vi "Add Item to Tree.vi"(8 "error in (no error)":errorcluster, 10 "Polymorphic VI Type in":refnum<class "Polymorphic VI Type.lvclass">, 11 "Tree Ref in":refnum<vi>) -> (0 "error out":errorcluster, 1 "Added Tag":string, 2 "Polymorphic VI Type out":refnum<class "Polymorphic VI Type.lvclass">, 3 "Tree Ref out":refnum<vi>)   [LabVIEW 2020, in "Peek Window.lvlib" / "Polymorphic VI Type.lvclass"]
uses:
  Polymorphic VI Type.lvclass
  D:/Code/VI-Peek/source/Peek Window/VI Types/Standard VI Type/Standard VI Type.lvclass
  Symbols Enum.ctl
  Standard VI Type/Standard VI Type.lvclass/Standard VI Type.ctl
  Standard VI Type/Read Full Qualified Name.vi
  Polymorphic VI Type.lvclass/Polymorphic VI Type.ctl
  Peek Window.lvlib
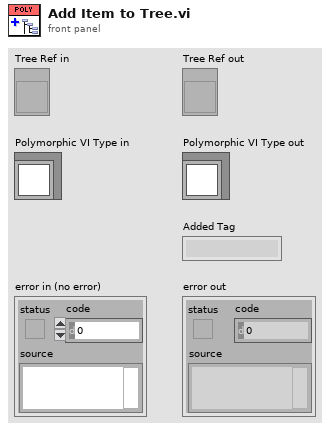
[diagram p1: front panel]
types:
  T1 = typedef "Peek Window.lvlib/Symbols Enum.ctl" = enum16{"<Blank>", "Below Here Glyph", "VI", "Dynamic Dispatch VI", "Malleable VI", "Polymorphic VI", "Missing VI", "Express VI"}
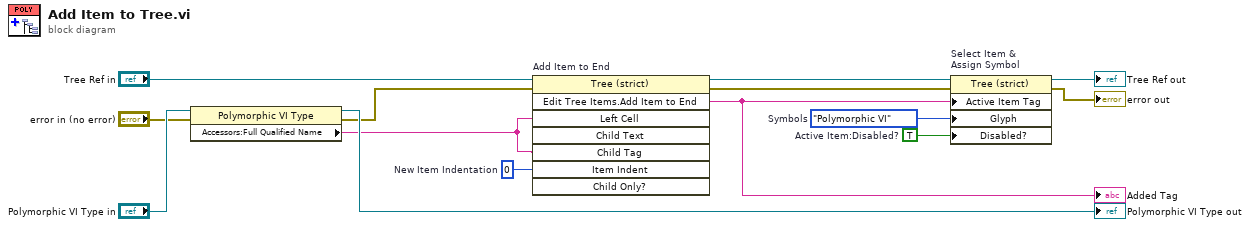
[diagram p0: block diagram]
diagram:
  w1 = TRUE  # Active Item:Disabled?
  w13 = Symbols_Enum."Polymorphic VI"  # Symbols
  w14 = 0  # New Item Indentation
  n1 = property class="Polymorphic VI Type"(reference="Polymorphic VI Type in", error in="error in (no error)") -> (reference out=→"Polymorphic VI Type out":refnum<class "Polymorphic VI Type.lvclass">, error out=w3:errorcluster, "Accessors:Full Qualified Name"=w2:string)
  n2 = invoke on="Add Item to End" class="Tree (strict)" method="Edit Tree Items.Add Item to End"(reference="Tree Ref in", error in=w3, "Left Cell"=w2, "Child Tag"=w2, "Item Indent"=w14) -> (reference out=w12:refnum<vi>, error out=w9:errorcluster, "Edit Tree Items:Add Item to End"=w7:string)  [unwired: 3 in, 5 out]
  "Added Tag" <- w7
  n3 = property on="Select Item &\nAssign Symbol" class="Tree (strict)"(reference=w12, error in=w9, "Active Item Tag"=w7, "Glyph"=w13, "Disabled?"=w1) -> (reference out=→"Tree Ref out":refnum<vi>, error out=→"error out":errorcluster)
